vi "__DVR API Template.vi"   [LabVIEW 2016, in "SLL Scripting.lvlib" / "SLL Class DVR API Generator.lvlib"]
uses:
  SLL Class DVR API Generator.lvlib
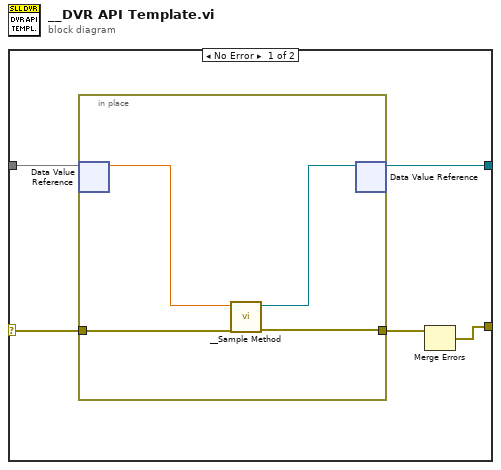
[diagram p0: block diagram]
diagram:
  n1 = case "Error Case Structure" shown="No Error" {
    selector: _ -> [w5 w11]
    tunnel: [w3 w11] -> _
    tunnel: [w2 w10] -> _
    tunnel: [w1 w10] -> _
    frame No Error {
      n2 = in-place "DVR In Place Element Structure" {
        in-place-border: w5 -> [w6]
        in-place-border: [w9] -> w4
        n3 = in-place-dvr #1(w2) -> (w8:dbl)  [unwired: 1 out]
        n4 = call "__Sample Method.vi"("error in (no error)"=w6, "My Sample Class in"=w8) -> ("error out"=w9:errorcluster, "My Sample Class out"=w7:refnum<class>)  [unwired: 8 in]
        n5 = in-place-dvr #1(w7) -> (w1:refnum<data-value>)  [unwired: 1 out]
      }
      n6 = Merge Errors(w4) -> (w3:errorcluster)  [unwired: 2 in]
    }
    frame Error {
    }
  }
